vi "0degDataView.vi"(0 "3 Column Array":dbl[][](array[numeric])) -> ()   [LabVIEW 2013]
panel:
  in  "stop":bool
  out "XY Graph":cluster{dbl[], dbl[]}(graph)
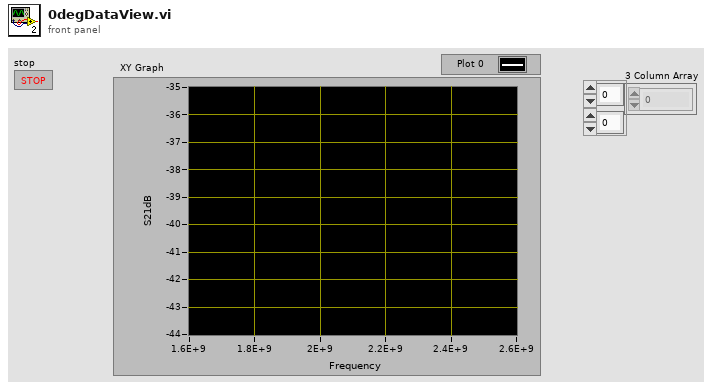
[diagram p1: front panel]
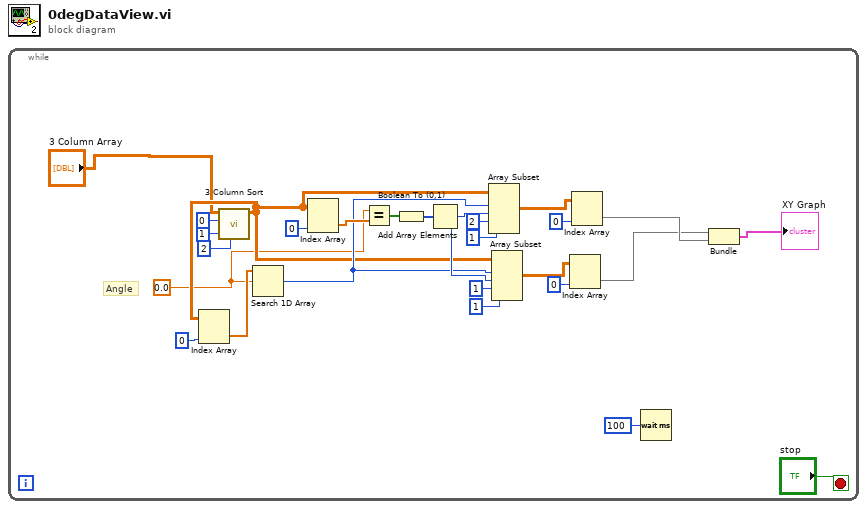
[diagram p0: block diagram]
diagram:
  n1 = while {
    stop <- "stop" stop-if-true
    w4 = 0.0 ("element")
    # "Angle"
    n2 = call "3 Column Sort.vi"("Tertiary Column"=2, "Secondary Column"=1, "Primary Column"=0, "3 Column Array"="3 Column Array") -> ("Sorted Array"=w6:dbl[][])  [unwired: 7 in]
    n3 = Index Array(array=w6, index (col)=0 ("disabled index (col)")) -> (element=w5:dbl[])  [unwired: 1 in]
    n4 = Search 1D Array(1D array=w5, element=w4) -> (index of element=w15:i32)  [unwired: 1 in]
    n5 = Index Array(array=w6, index (col)=0 ("disabled index (col)")) -> (element=w25:dbl[])  [unwired: 1 in]
    n6 = Equal?(x=w4, y=w25) -> (x = y?=w24:bool[])
    n7 = Boolean To (0,1)(Boolean=w24) -> (0, 1=w27:i16[])
    n8 = Add Array Elements(numeric array=w27) -> (sum=w16:i16)
    n9 = Array Subset(array=w6, index (row)=w15, length (row)=w16, index (col)=2 ("index"), length (col)=1 ("length")) -> (w14:dbl[][])
    n10 = Array Subset(array=w6, index (row)=w15, length (row)=w16, index (col)=1 ("index"), length (col)=1 ("length")) -> (w13:dbl[][])
    n11 = Index Array(array=w13, index (col)=0 ("disabled index (col)")) -> (element=w8:dbl[])  [unwired: 1 in]
    n12 = Index Array(array=w14, index (col)=0 ("disabled index (col)")) -> (element=w9:dbl[])  [unwired: 1 in]
    n13 = Wait (ms)(milliseconds to wait=u32 100) -> ()  [unwired: 1 out]
    n14 = Bundle(w8, w9) -> (→"XY Graph":cluster{dbl[], dbl[]})  [unwired: 1 in]
  }
